vi "Read Attributes.vi"(11 "PS Dataset Msg":refnum<class "PS Dataset Msg.lvclass">) -> (2 "Payload":T1)   [LabVIEW 2019, in "Power Supply.lvlib" / "PS Dataset Msg.lvclass"]
uses:
  PS Dataset Msg.lvclass
  PS Dataset Msg.lvclass/PS Dataset Msg.ctl
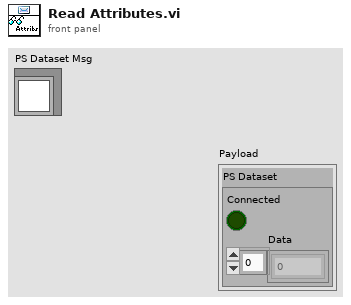
[diagram p1: front panel]
types:
  T1 = cluster{"PS Dataset":cluster{"Connected":bool, "Data":dbl[]}}
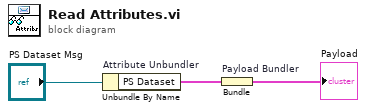
[diagram p0: block diagram]
diagram:
  n1 = Unbundle By Name "Attribute Unbundler"("PS Dataset Msg") -> ("PS Dataset"=w1:cluster{"Connected":bool, "Data":dbl[]})
  n2 = Bundle "Payload Bundler"("PS Dataset"=w1) -> (→"Payload":T1)  [unwired: 1 in]
